vi "ScansteuerungDisplayImageFromScan.vi"(1 "Linear conversion Matrix":dbl[][](array[numeric]), 2 "Imagesize [Pixel]":cluster{"width":u32, "height":u32}={"width"=500, "height"=500}, 3 "ScanSteuerung":T2(array[cluster])=[{"Zeitpunkt [s]"=0.0, "Wirkung"=enum."Abs", "Kanal"=enum."SMoveTime", "Wert (/s)"=0.00119}, {"Zeitpunkt [s]"=0.0, "Wirkung"=enum."Abs", "Kanal"=enum."GalvoX", "Wert (/s)"=-0.001005733}, {"Zeitpunkt [s]"=0.0, "Wirkung"=enum."Abs", "Kanal"=enum."GalvoY", "Wert (/s)"=0.0012455387}, {"Zeitpunkt [s]"=0.0, "Wirkung"=enum."Abs", "Kanal"=enum."Image1X", "Wert (/s)"=0.0}, {"Zeitpunkt [s]"=0.0, "Wirkung"=enum."Abs", "Kanal"=enum."Image1Y", "Wert (/s)"=0.0}, {"Zeitpunkt [s]"=0.0, "Wirkung"=enum."Abs", "Kanal"=enum."Digital", "Wert (/s)"=7.0}, {"Zeitpunkt [s]"=0.0, "Wirkung"=enum."LoopStart", "Kanal"=enum."Loop", "Wert (/s)"=399.0}, {"Zeitpunkt [s]"=0.0, "Wirkung"=enum."Inc", "Kanal"=enum."GalvoX", "Wert (/s)"=1.966139951}, {"Zeitpunkt [s]"=0.0, "Wirkung"=enum."Inc", "Kanal"=enum."GalvoY", "Wert (/s)"=-0.5873650426}, {"Zeitpunkt [s]"=0.0, "Wirkung"=enum."IncInc", "Kanal"=enum."GalvoX", "Wert (/s)"=0.0}, {"Zeitpunkt [s]"=0.0, "Wirkung"=enum."IncInc", "Kanal"=enum."GalvoY", "Wert (/s)"=0.0}, {"Zeitpunkt [s]"=0.0, "Wirkung"=enum."Inc", "Kanal"=enum."Image1X", "Wert (/s)"=200000.0}, {"Zeitpunkt [s]"=0.001995, "Wirkung"=enum."Inc", "Kanal"=enum."Image1X", "Wert (/s)"=0.0}, {"Zeitpunkt [s]"=0.002, "Wirkung"=enum."Inc", "Kanal"=enum."Image1X", "Wert (/s)"=-1564705.8823529398}, {"Zeitpunkt [s]"=0.002, "Wirkung"=enum."Rel", "Kanal"=enum."Image1Y", "Wert (/s)"=1.0}, {"Zeitpunkt [s]"=0.002, "Wirkung"=enum."Abs", "Kanal"=enum."Digital", "Wert (/s)"=5.0}, {"Zeitpunkt [s]"=0.002, "Wirkung"=enum."IncInc", "Kanal"=enum."GalvoX", "Wert (/s)"=-263085.1079131726}, {"Zeitpunkt [s]"=0.002, "Wirkung"=enum."IncInc", "Kanal"=enum."GalvoY", "Wert (/s)"=78019.7708861241}, {"Zeitpunkt [s]"=0.00213, "Wirkung"=enum."IncInc", "Kanal"=enum."GalvoX", "Wert (/s)"=263085.1079131726}, {"Zeitpunkt [s]"=0.00213, "Wirkung"=enum."IncInc", "Kanal"=enum."GalvoY", "Wert (/s)"=-78019.7708861241}, {"Zeitpunkt [s]"=0.002255, "Wirkung"=enum."Inc", "Kanal"=enum."Image1X", "Wert (/s)"=0.0}, {"Zeitpunkt [s]"=0.00226, "Wirkung"=enum."Abs", "Kanal"=enum."Digital", "Wert (/s)"=7.0}, {"Zeitpunkt [s]"=0.00226, "Wirkung"=enum."LoopEnd", "Kanal"=enum."Loop", "Wert (/s)"=0.0}, {"Zeitpunkt [s]"=0.90174, "Wirkung"=enum."Inc", "Kanal"=enum."GalvoX", "Wert (/s)"=1.966139951}, {"Zeitpunkt [s]"=0.90174, "Wirkung"=enum."Inc", "Kanal"=enum."GalvoY", "Wert (/s)"=-0.5873650426}, {"Zeitpunkt [s]"=0.90174, "Wirkung"=enum."IncInc", "Kanal"=enum."GalvoX", "Wert (/s)"=0.0}, {"Zeitpunkt [s]"=0.90174, "Wirkung"=enum."IncInc", "Kanal"=enum."GalvoY", "Wert (/s)"=0.0}, {"Zeitpunkt [s]"=0.90174, "Wirkung"=enum."Inc", "Kanal"=enum."Image1X", "Wert (/s)"=200000.0}, {"Zeitpunkt [s]"=0.903735, "Wirkung"=enum."Inc", "Kanal"=enum."Image1X", "Wert (/s)"=0.0}, {"Zeitpunkt [s]"=0.90374, "Wirkung"=enum."Inc", "Kanal"=enum."GalvoX", "Wert (/s)"=0.0}, {"Zeitpunkt [s]"=0.90374, "Wirkung"=enum."Inc", "Kanal"=enum."GalvoY", "Wert (/s)"=0.0}, {"Zeitpunkt [s]"=0.90374, "Wirkung"=enum."Abs", "Kanal"=enum."Digital", "Wert (/s)"=0.0}], 4 "Intensity Graph":i16[][](graph)=array400x400[160000 elements]) -> (5 "PixmapBild":i16[][](graph))   [LabVIEW 2011]
panel:
  in  "Sorry need Galvo-clock":dbl=1e-05
  out "Sampled pixels":i32=180748
  out "size(s)":i32=90375
  out "Pixelcycle":dbl=5e-06 min=0.4 max=10000.0 step=0.05
  out "Galvo-cycle":dbl=1e-05
  out "XY Graph-Pixels!":T1(graph)
  # "Alt:\ngeht nur für Loops= festes Zeilenincrement, da das Zeilenincrement für die \"höhe\" des streifens benötigt wird\nman könnte höchstens mit einem \"Airy-unit\" dicken \"Stift\" malen, ist aber ein ganz anderes Modul"
  # "Geht gut!\nwenn loop da: Breite=Zeilenabstand\nsonst ~2pixel hoch?!"
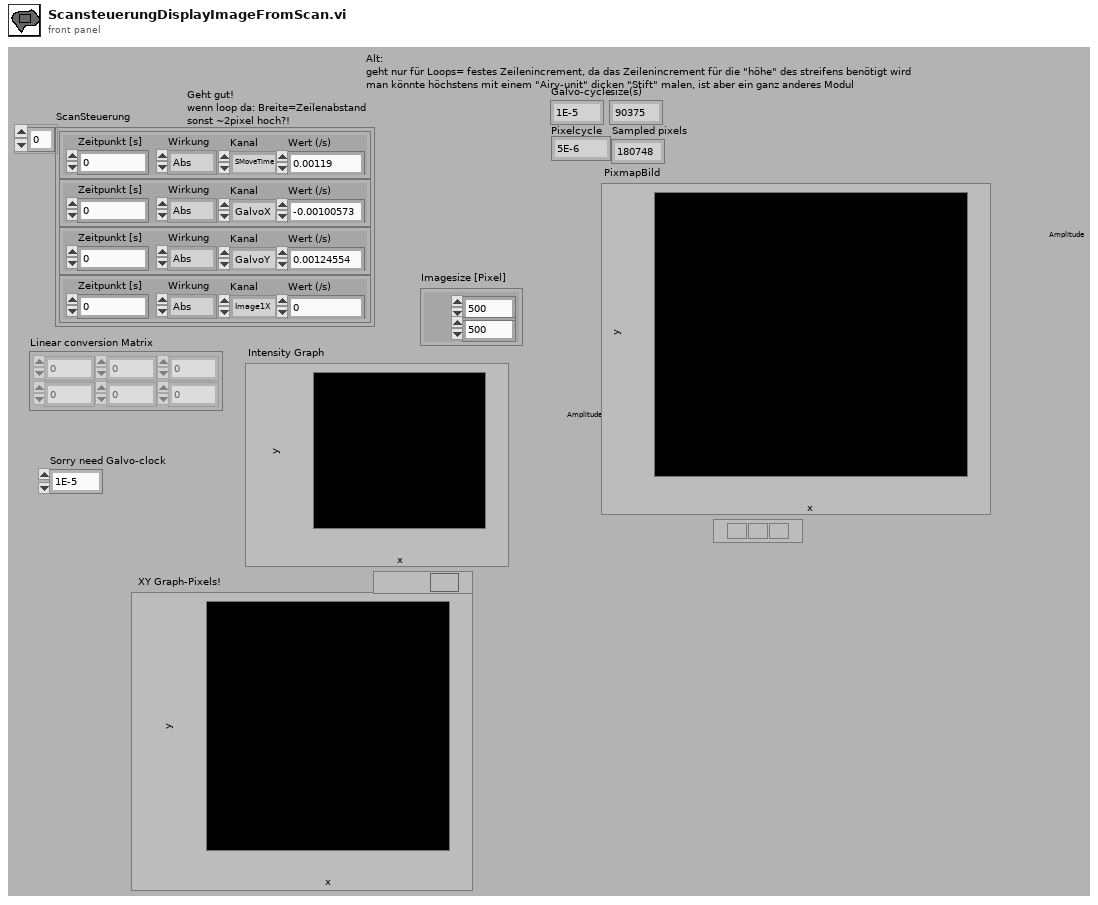
[diagram p1: front panel]
types:
  T1 = cluster{"number: 0 to 1":dbl, "number: 0 to 1":dbl}[]
  T2 = cluster{"Zeitpunkt [s]":dbl, "Wirkung":enum16{"Abs", "Rel", "Inc", "IncInc", "LoopStart", "LoopEnd"}, "Kanal":enum16{"Com", "AnalogConfig", "AnalogValue", "GalvoX", "GalvoY", "Galvo3", "Galvo4", "Digital", "Free", "Loop", "SMoveTime", "Image1X", "Image1Y", "Image2X", "Image2Y"}, "Wert (/s)":dbl}[]
  T3 = enum16{"Com", "AnalogConfig", "AnalogValue", "GalvoX", "GalvoY", "Galvo3", "Galvo4", "Digital", "Free", "Loop", "SMoveTime", "Image1X", "Image1Y", "Image2X", "Image2Y"}[]
  T4 = cluster{"Waveform Graph[0]":dbl, "Waveform Graph[1]":dbl}
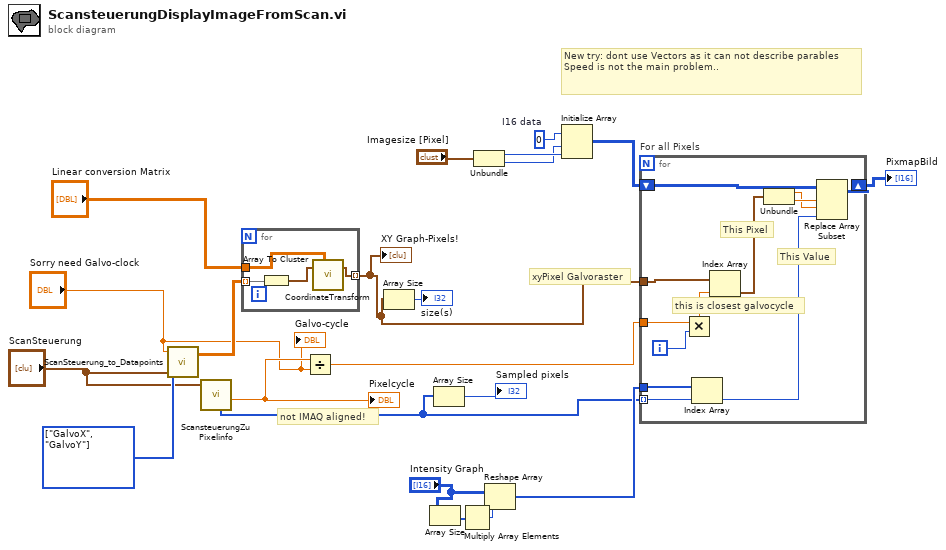
[diagram p0: block diagram]
diagram:
  w13 = T3 [enum."GalvoX", enum."GalvoY"] items=["Com", "AnalogConfig", "AnalogValue", "GalvoX", "GalvoY", "Galvo3", "Galvo4", "Digital", "Free", "Loop", "SMoveTime", "Image1X", "Image1Y", "Image2X", "Image2Y"] ("Aktiv")
  w21 = i16 0  # I16 data
  # "not IMAQ aligned!"
  # "New try: dont use Vectors as it can not describe parables\nSpeed is not the main problem.."
  # "xyPixel Galvoraster"
  n1 = call "ScanSteuerung_to_Datapoints.vi"("ScanSteuerung"="ScanSteuerung", "Aktiv"=w13, "Neues Zeitraster"="Sorry need Galvo-clock") -> ("Waveform Graph"=w12:dbl[][])  [unwired: 1 in, 1 out]
  n2 = call "ScansteuerungZuPixelinfo.vi"("ScanSteuerung"="ScanSteuerung") -> ("Pixelindex"=w4:u32[], "Pixelzeit in s"=w8:dbl)  [unwired: 1 in, 5 out]
  "Pixelcycle" <- w8
  n3 = for {
    tunnel: "Linear conversion Matrix" -> [w22]
    tunnel: w12 -> [w25] mode=indexing
    tunnel: [w23] -> w9 mode=indexing
    n4 = Array To Cluster(array=w25) -> (cluster=w24:T4)
    n5 = call "CoordinateTransform.vi"("input coordiantes"=w24, "Conversion Matrix"=w22) -> ("output coordiantes"=w23:cluster{"x":dbl, "y":dbl})  [unwired: 2 in, 1 out]
  }
  "XY Graph-Pixels!" <- w9
  n6 = Divide(x=w8, y="Sorry need Galvo-clock") -> (x/y=w6:dbl)
  n7 = Array Size(array=w9) -> (size(s)=→"size(s)":i32)
  n8 = Array Size(array="Intensity Graph") -> (size(s)=w18:i32[])
  n9 = Array Size(array=w4) -> (size(s)=→"Sampled pixels":i32)
  n10 = Multiply Array Elements(1:w18) -> (0:w17:i32)
  n11 = Unbundle("Imagesize [Pixel]") -> ("width"=w15:u32, "height"=w14:u32)
  n12 = Reshape Array("Intensity Graph", w17) -> (w10:i16[])
  n13 = Initialize Array(w21, w14, w15) -> (w11:i16[][])
  n14 = for "For all Pixels" {
    shift-right: [w37] -> w16
    shift-left: w11 -> [w36]
    tunnel: w10 -> [w34]
    tunnel: w4 -> [w29] mode=indexing
    tunnel: w9 -> [w33]
    tunnel: w6 -> [w32]
    i -> [w31]
    # "this is closest galvocycle"
    # "This Value"
    # "This Pixel"
    n15 = Multiply(x=w32, y=w31) -> (x*y=w30:dbl)
    n16 = Index Array(array=w34, index=w29) -> (element=w35:i16)
    n17 = Index Array(array=w33, index=w30) -> (element=w28:cluster{"x":dbl, "y":dbl})
    n18 = Unbundle(w28) -> ("x"=w26:dbl, "y"=w27:dbl)
    n19 = Replace Array Subset(array=w36, new element=w35, index (row)=w27, index (col)=w26) -> (w37:i16[][])
  }
  "PixmapBild" <- w16
  "Galvo-cycle" <- "Sorry need Galvo-clock"
